vi "BuildMsg.vi"(7 "Data":u8[](array[numeric]), 8 "error in":errorcluster, 9 "HostAddress":u8, 10 "UnitAddress":u8, 11 "TxID":u32) -> (0 "error out":errorcluster, 3 "MsgTX 2":T1)   [LabVIEW 2017]
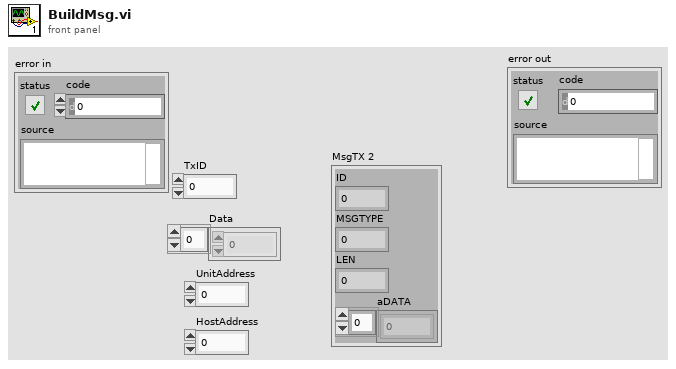
[diagram p1: front panel]
types:
  T1 = cluster{"ID":u32, "MSGTYPE":u8, "LEN":u8, "aDATA":u8[]}
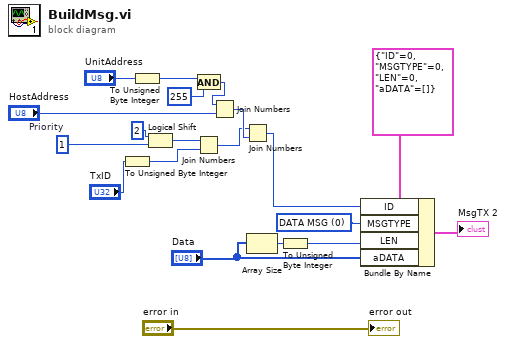
[diagram p0: block diagram]
diagram:
  w4 = u8 1  # Priority
  w20 = u8 0 items=["STATUS"=128, "EXTENDED"=2, "RTR"=1, "DATA MSG"=0] ("MSGTYPE")
  n1 = To Unsigned Byte Integer(number="TxID") -> (unsigned 8bit integer=w5:u8)
  n2 = To Unsigned Byte Integer(number="UnitAddress") -> (unsigned 8bit integer=w10:u8)
  n3 = Logical Shift(y=u8 2, x=w4) -> (x << y=w6:u8)
  n4 = And(x=w10, y=u8 255) -> (x .and. y?=w8:u8)
  n5 = Join Numbers(hi=w6, lo=w5) -> ((hi.lo)=w13:u16)
  n6 = Join Numbers(hi=w8, lo="HostAddress") -> ((hi.lo)=w14:u16)
  n7 = Join Numbers(hi=w13, lo=w14) -> ((hi.lo)=w11:u32)
  n8 = Array Size(array="Data") -> (size(s)=w16:i32)
  n9 = To Unsigned Byte Integer(number=w16) -> (unsigned 8bit integer=w19:u8)
  n10 = Bundle By Name(cluster=T1 {"ID"=0, "MSGTYPE"=0, "LEN"=0, "aDATA"=[]} ("MsgTX 2"), "ID"=w11, "MSGTYPE"=w20, "LEN"=w19, "aDATA"="Data") -> (→"MsgTX 2":T1)
  "error out" <- "error in"
